vi "Open Logs.vi"(8 "error in":errorcluster, 11 "Fault Handler in":refnum<class "Fault Handler.lvclass">) -> (0 "error out":errorcluster, 3 "Fault Handler out":refnum<class "Fault Handler.lvclass">)   [LabVIEW 2023, in "Fault Handler.lvlib" / "Fault Handler.lvclass"]
uses:
  Library/Fault Handler.lvclass
  C:/Users/Public/Documents/Development/builds/Engine/Engine.lvlibp/Project/Engine.lvclass
  Library/Fault Handler.lvclass/Fault Handler.ctl
  builds/Engine/Engine.lvlibp/Accessors/Read Directory.vi
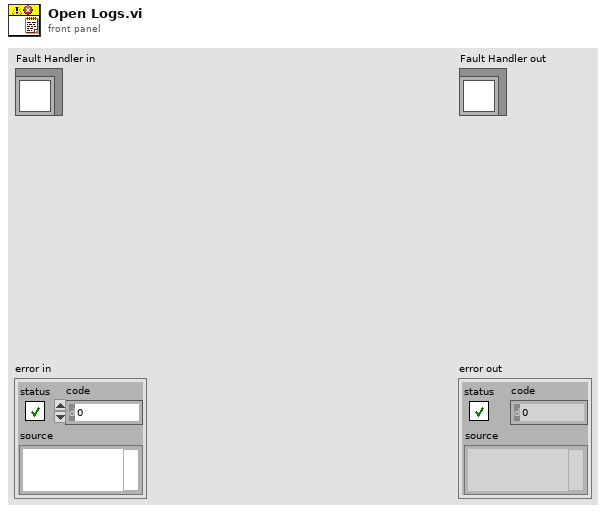
[diagram p1: front panel]
types:
  T1 = enum16{"open", "replace", "create", "open or create", "replace or create", "replace or create with confirmation"}
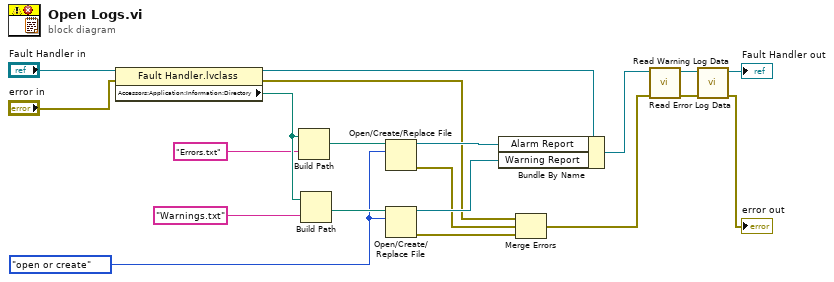
[diagram p0: block diagram]
diagram:
  w13 = T1."open or create" ("operation (0:open)")
  n1 = property class="Fault Handler.lvclass"(reference="Fault Handler in", error in="error in") -> (reference out=w12:refnum<class "Fault Handler.lvclass">, error out=w9:errorcluster, "Accessors:Application:Information:Directory"=w18:path)
  n2 = Build Path(base path=w18, name or relative path="Errors.txt") -> (appended path=w15:path)
  n3 = Build Path(base path=w18, name or relative path="Warnings.txt") -> (appended path=w14:path)
  n4 = Open/Create/Replace File(file path (use dialog)=w15, operation (0:open)=w13) -> (refnum out=w11:refnum<file>, error out=w8:errorcluster)  [unwired: 4 in, 1 out]
  n5 = Open/Create/Replace File(file path (use dialog)=w14, operation (0:open)=w13) -> (refnum out=w10:refnum<file>, error out=w7:errorcluster)  [unwired: 4 in, 1 out]
  n6 = Bundle By Name(cluster=w12, "Alarm Report"=w11, "Warning Report"=w10) -> (w4:refnum<class "Fault Handler.lvclass">)
  n7 = Merge Errors(w9, w8, w7) -> (w3:errorcluster)
  n8 = call "Read Error Log Data.vi"("error in"=w3, "Fault Handler in"=w4) -> ("error out"=w6:errorcluster, "Fault Handler out"=w5:refnum<class "Fault Handler.lvclass">)  [unwired: 8 in]
  n9 = call "Read Warning Log Data.vi"("error in"=w6, "Fault Handler in"=w5) -> ("error out"=→"error out":errorcluster, "Fault Handler out"=→"Fault Handler out":refnum<class "Fault Handler.lvclass">)  [unwired: 8 in]
